vi "resultsColumnsPWA.vi"(10 "chValuesIn":string[](array[string]), 11 "chNamesIn":string[](array[string])) -> (2 "chValuesOut":string[](array[string]), 3 "chNamesOut":string[](array[string]))   [LabVIEW 2020]
uses:
  Acquisition/PWA/PWAtasksGLOBAL.vi
  Globals/Meas_global.vi
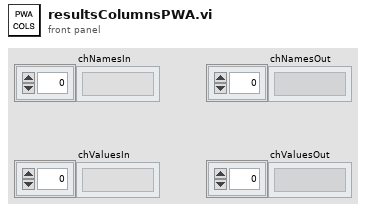
[diagram p1: front panel]
types:
  T1 = typedef "PWA_Data.ctl" = enum16{"No PWA Data", "One Ch PWA"}
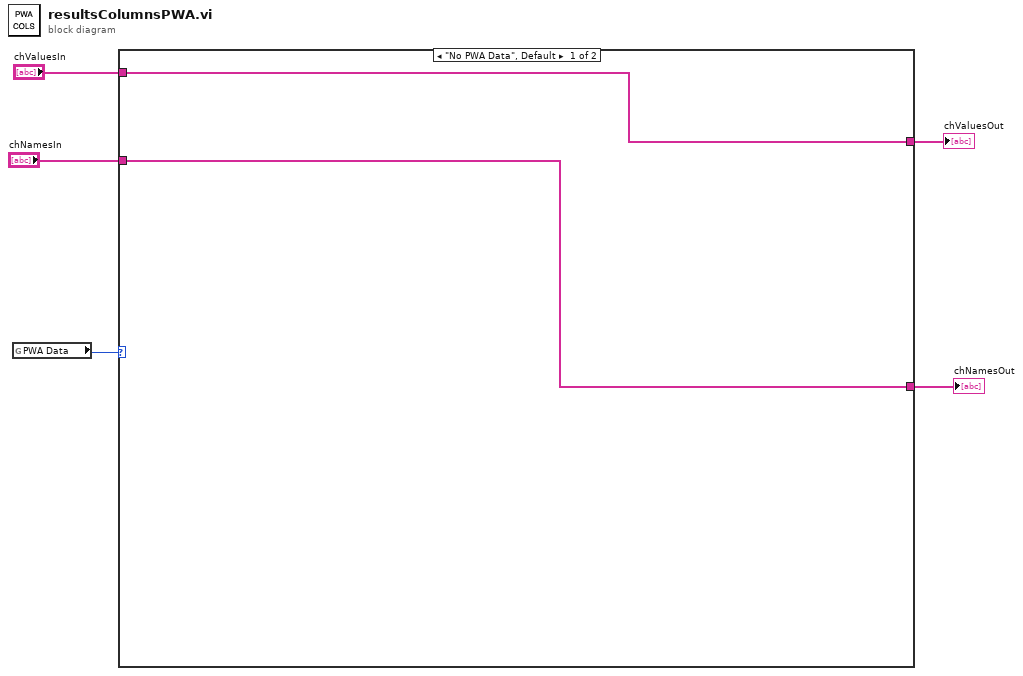
[diagram p0: block diagram]
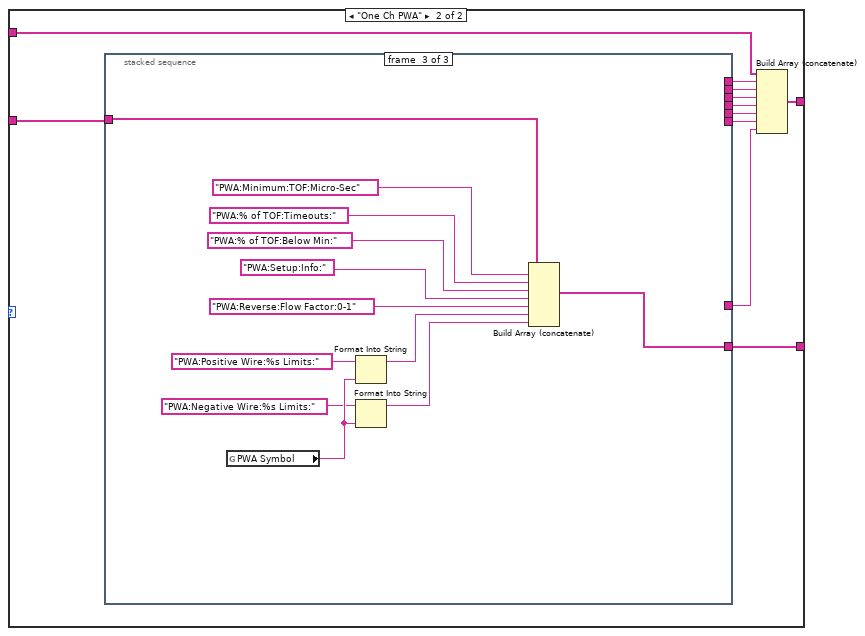
[diagram p2: hidden frame]
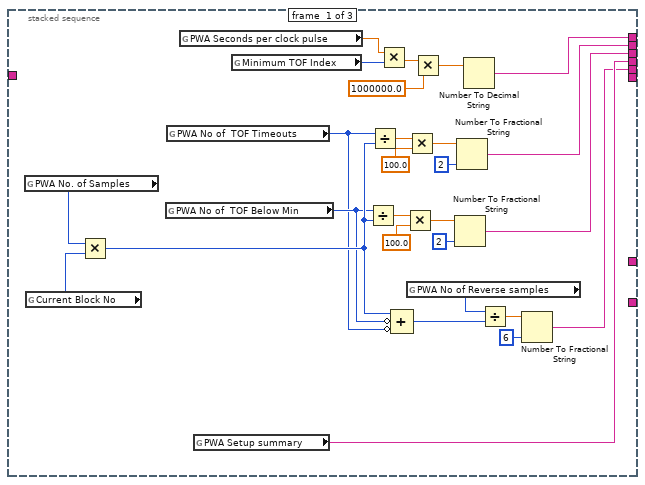
[diagram p3: hidden frame]
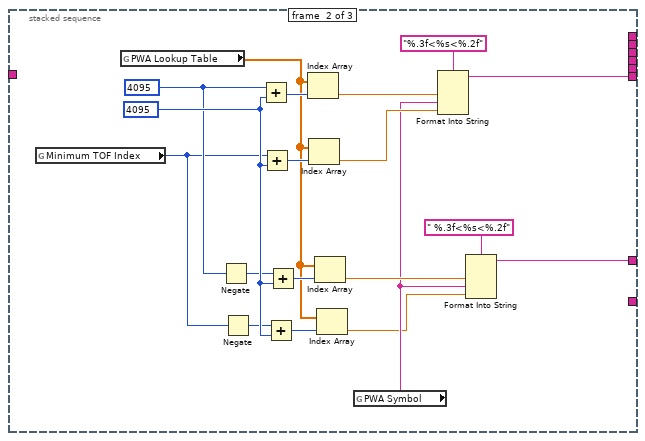
[diagram p4: hidden frame]
diagram:
  n1 = global read "Meas_global.vi" "PWA Data"() -> (w1:T1)
  n2 = case shown="\"No PWA Data\", Default" w1 {
    tunnel: "chValuesIn" -> [w7 w18]
    tunnel: [w6 w17] -> w4
    tunnel: "chNamesIn" -> [w6 w16]
    tunnel: [w7 w8] -> w2
    frame "No PWA Data", Default {
    }
    frame "One Ch PWA" {
      n3 = stacked-sequence {
        tunnel: [w40 _ _] -> w9
        tunnel: [w35 _ _] -> w10
        tunnel: [w34 _ _] -> w11
        tunnel: [_ w47 _] -> w12
        tunnel: [_ w46 _] -> w13
        tunnel: [w28 _ _] -> w14
        tunnel: [w20 _ _] -> w15
        tunnel: w16 -> [_ _ w66]
        tunnel: [_ _ w65] -> w17
        frame #0 {
          n4 = global read "PWAtasksGLOBAL.vi" "PWA No. of Samples"() -> (w45:i32)
          n5 = global read "Meas_global.vi" "Current Block No"() -> (w19:i32)
          n6 = Multiply(x=w45, y=w19) -> (x*y=w27:i32)
          n7 = global read "PWAtasksGLOBAL.vi" "PWA No of  TOF Below Min"() -> (w26:i32)
          n8 = global read "PWAtasksGLOBAL.vi" "PWA No of  TOF Timeouts"() -> (w25:i32)
          n9 = global read "PWAtasksGLOBAL.vi" "PWA Seconds per clock pulse"() -> (w32:dbl)
          n10 = global read "PWAtasksGLOBAL.vi" "PWA Setup summary"() -> (w34:string)
          n11 = global read "PWAtasksGLOBAL.vi" "Minimum TOF Index"() -> (w33:i16)
          n12 = Divide(x=w26, y=w27) -> (x/y=w36:dbl)
          n13 = Divide(x=w25, y=w27) -> (x/y=w44:dbl)
          n14 = Multiply(x=w32, y=w33) -> (x*y=w31:dbl)
          n15 = Compound Arithmetic op=ADD(w27, invert w26, invert w25) -> (w23:i32)
          n16 = Multiply(x=w36, y=100.0) -> (x*y=w39:dbl)
          n17 = Multiply(x=w44, y=100.0) -> (x*y=w41:dbl)
          n18 = global read "PWAtasksGLOBAL.vi" "PWA No of Reverse samples"() -> (w24:i32)
          n19 = Multiply(x=w31, y=1000000.0) -> (x*y=w29:dbl)
          n20 = Number To Fractional String(number=w39, precision (6)=i16 2) -> (F-format string=w35:string)  [unwired: 2 out]
          n21 = Number To Fractional String(number=w41, precision (6)=i16 2) -> (F-format string=w40:string)  [unwired: 2 out]
          n22 = Number To Decimal String(number=w29) -> (decimal integer string=w28:string)  [unwired: 1 out]
          n23 = Divide(x=w24, y=w23) -> (x/y=w21:dbl)
          n24 = Number To Fractional String(number=w21, precision (6)=i16 6) -> (F-format string=w20:string)  [unwired: 2 out]
        }
        frame #1 {
          w60 = 4095
          w56 = 4095
          n25 = global read "PWAtasksGLOBAL.vi" "Minimum TOF Index"() -> (w55:i16)
          n26 = global read "PWAtasksGLOBAL.vi" "PWA Lookup Table"() -> (w59:dbl[])
          n27 = Negate(x=w56) -> (-x=w58:i32)
          n28 = Negate(x=w55) -> (-x=w57:i16)
          n29 = Add(x=w56, y=w60) -> (x+y=w61:i32)
          n30 = Add(x=w55, y=w60) -> (x+y=w62:i32)
          n31 = Add(x=w57, y=w60) -> (x+y=w64:i32)
          n32 = Add(x=w58, y=w60) -> (x+y=w63:i32)
          n33 = Index Array(array=w59, index=w61) -> (element=w54:dbl)
          n34 = Index Array(array=w59, index=w62) -> (element=w53:dbl)
          n35 = Index Array(array=w59, index=w63) -> (element=w50:dbl)
          n36 = Index Array(array=w59, index=w64) -> (element=w48:dbl)
          n37 = global read "PWAtasksGLOBAL.vi" "PWA Symbol"() -> (w49:string)
          n38 = Format Into String(format string="%.3f<%s<%.2f", w54, w49, w53) -> (resulting string=w47:string)  [unwired: 2 in, 1 out]
          n39 = Format Into String(format string=" %.3f<%s<%.2f", w50, w49, w48) -> (resulting string=w46:string)  [unwired: 2 in, 1 out]
        }
        frame #2 {
          n40 = global read "PWAtasksGLOBAL.vi" "PWA Symbol"() -> (w69:string)
          n41 = Format Into String(format string="PWA:Positive Wire:%s Limits:", w69) -> (resulting string=w73:string)  [unwired: 2 in, 1 out]
          n42 = Format Into String(format string="PWA:Negative Wire:%s Limits:", w69) -> (resulting string=w74:string)  [unwired: 2 in, 1 out]
          n43 = Build Array (concatenate)(w66, "PWA:Minimum:TOF:Micro-Sec", "PWA:% of TOF:Timeouts:", "PWA:% of TOF:Below Min:", "PWA:Setup:Info:", "PWA:Reverse:Flow Factor:0-1", w73, w74) -> (w65:string[])
        }
      }
      n44 = Build Array (concatenate)(w18, w14, w9, w10, w11, w15, w12, w13) -> (w8:string[])
    }
  }
  "chNamesOut" <- w4
  "chValuesOut" <- w2
